vi "TCP Multiple Connections - Server.vi"() -> ()   [LabVIEW 2011]
doc: "This is the TCP server VI that supports multiple connections from client VIs."
panel:
  in  "Stop":bool
  out "Current Data":dbl
  out "# of Connections":i32
  # "Overview: Demonstrates the use of the TCP functions to initialize a TCP server that can send data to multiple client VIs.\nInstructions:\n1. Run the VI.\n2. Open TCP Multiple Connections - Client 1.vi and follow the instructions on its front panel.\n3. Open TCP Multiple Connections - Client 2.vi and follow the instructions on its front panel.\n4. Click Stop to stop the VI."
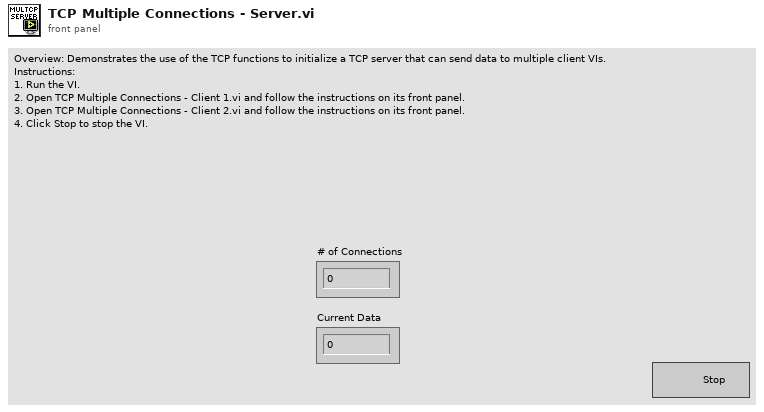
[diagram p1: front panel]
types:
  T1 = cluster{"Clients":refnum<k5>[], "Listener":refnum<k5>}
  T2 = enum16{"Initialize", "Status Check", "Send Data", "Stop"}
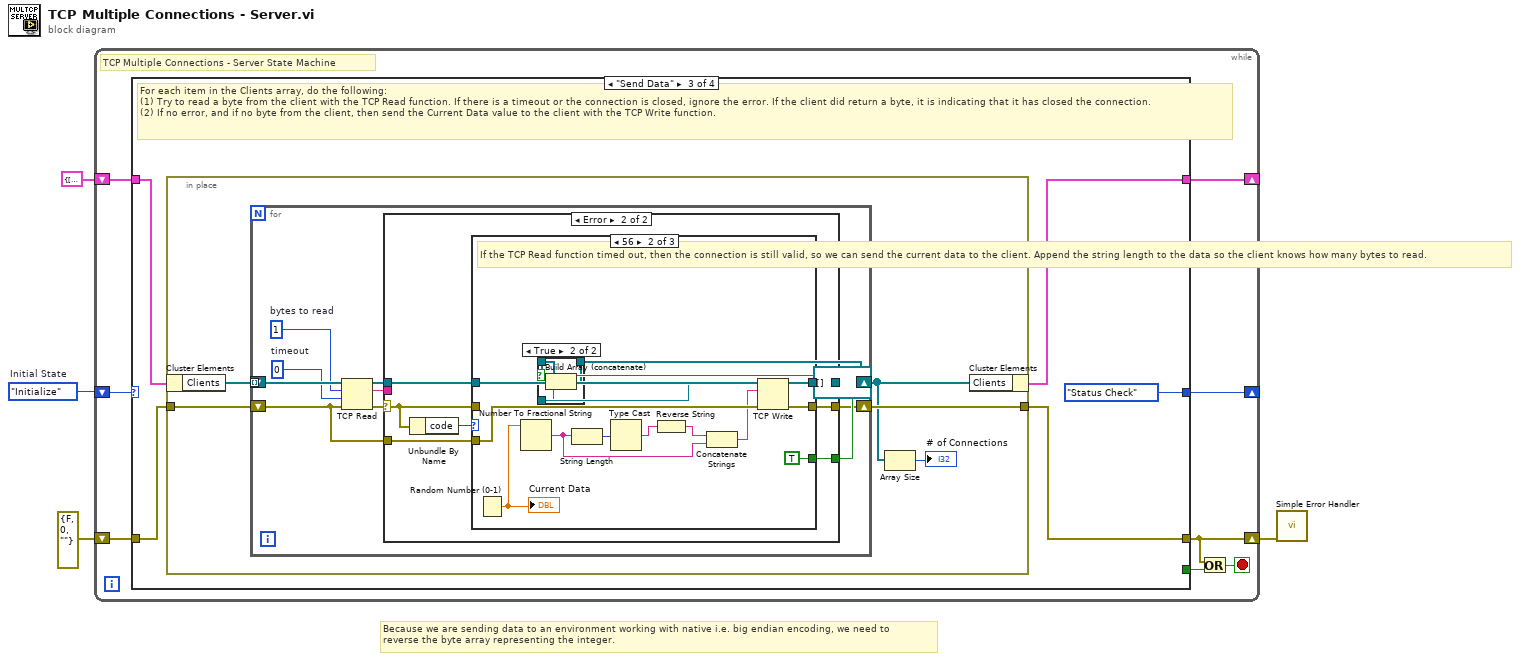
[diagram p0: block diagram]
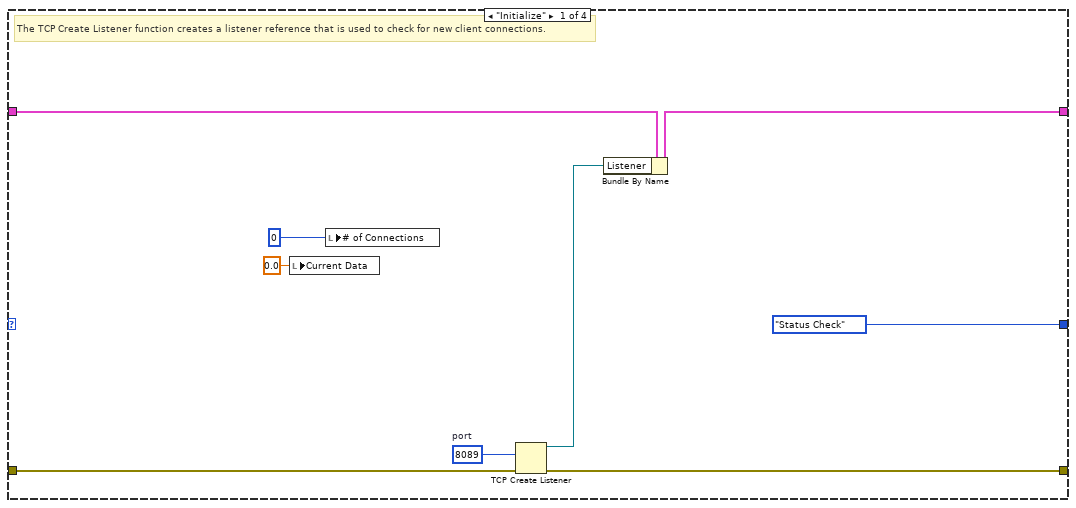
[diagram p2: hidden frame]
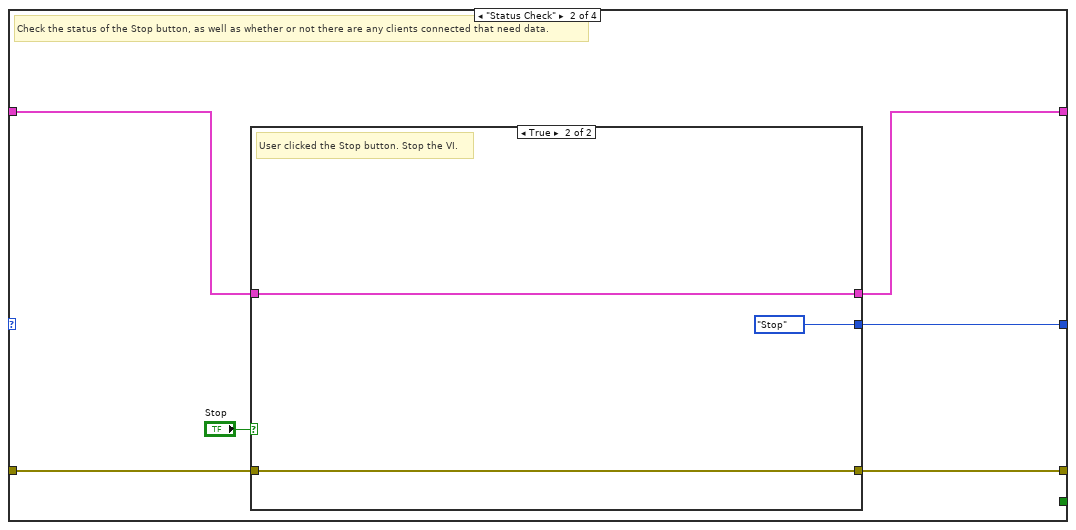
[diagram p3: hidden frame]
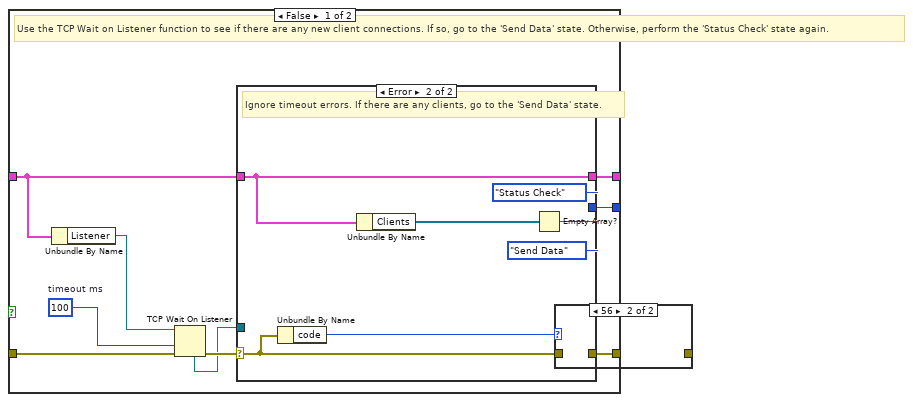
[diagram p4: hidden frame]
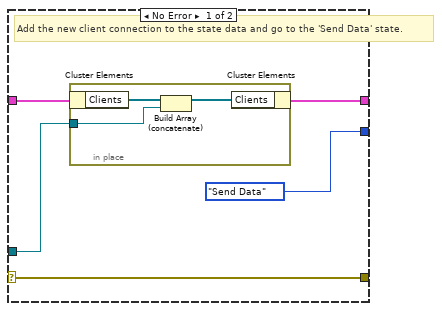
[diagram p5: hidden frame]
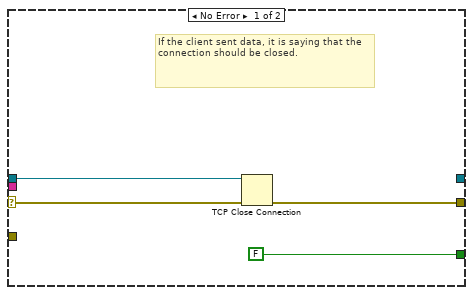
[diagram p8: hidden frame]
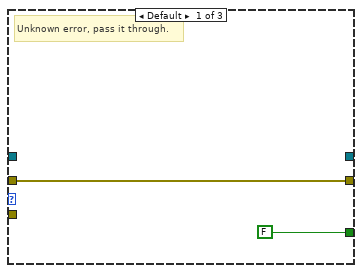
[diagram p9: hidden frame]
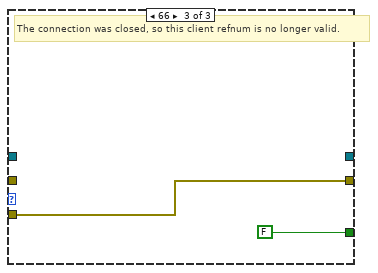
[diagram p10: hidden frame]
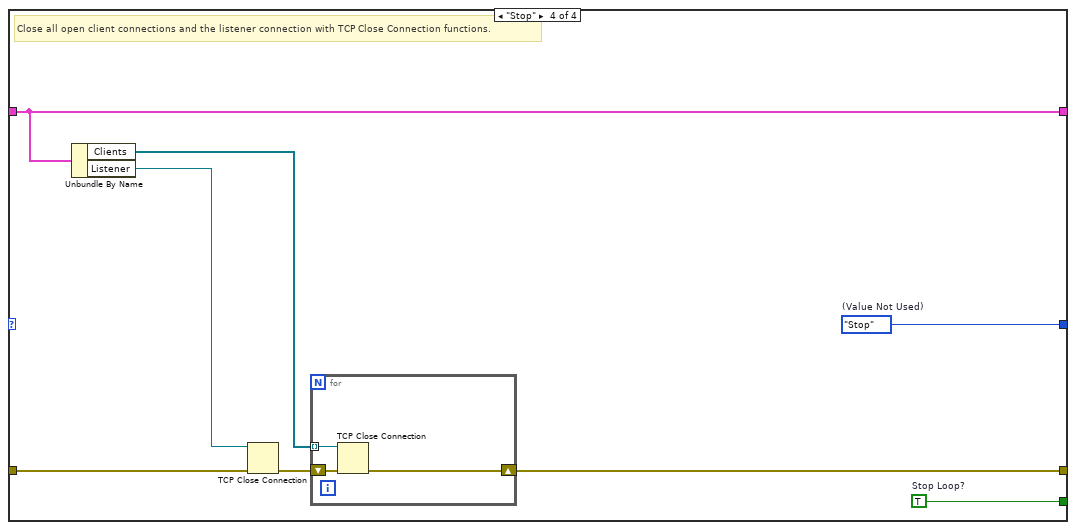
[diagram p11: hidden frame]
diagram:
  w4 = T2."Initialize"  # Initial State
  # "Because we are sending data to an environment working with native i.e. big endian encoding, we need to\nreverse the byte array representing the integer."
  n1 = while {
    shift-right: [w11] -> _
    shift-left: w4 -> [w12]
    shift-right: [w9] -> _
    shift-left: T1 {"Clients"=[], "Listener"=refnum} ("Data") -> [w10]
    shift-right: [w5] -> w1
    shift-left: errorcluster {"status"=FALSE, "code"=0, "source"=""} ("error constant") -> [w8]
    stop <- w6 stop-if-true
    # "TCP Multiple Connections - Server State Machine"
    n2 = case shown="\"Send Data\"" w12 {
      tunnel: [T2."Status Check" ("States") w27 T2."Status Check" ("States") w112] -> w11
      tunnel: [_ _ _ w119] -> w7
      tunnel: w10 -> [w19 w23 w61 w118]
      tunnel: [w18 w22 w60 w118] -> w9
      tunnel: w8 -> [w21 w26 w63 w117]
      tunnel: [w20 w25 w62 w115] -> w5
      frame "Initialize" {
        w16 = u16 8089  # port
        # "The TCP Create Listener function creates a listener reference that is used to check for new client connections."
        n3 = local write "Current Data"(0.0 ("Current Data")) -> ()
        n4 = local write "# of Connections"(0 ("Number of Client Connections")) -> ()
        n5 = TCP Create Listener(8:w21, 10:w16) -> (0:w20:errorcluster, 3:w17:refnum<k5>)  [unwired: 4 out]
        n6 = Bundle By Name(cluster=w19, "Listener"=w17) -> (w18:T1)
      }
      frame "Status Check" {
        # "Check the status of the Stop button, as well as whether or not there are any clients connected that need data."
        n7 = case shown="True" "Stop" {
          tunnel: [w36 T2."Stop" ("States")] -> w27
          tunnel: w26 -> [w35 w58]
          tunnel: [w28 w58] -> w25
          tunnel: w23 -> [w31 w57]
          tunnel: [w30 w57] -> w22
          frame False {
            w34 = 100  # timeout ms
            # "Use the TCP Wait on Listener function to see if there are any new client connections. If so, go to the 'Send Data' state. Otherwise, perform the 'Status Check' state again."
            n8 = Unbundle By Name(w31) -> ("Listener"=w29:refnum<k5>)
            n9 = TCP Wait On Listener(8:w35, 9:w34, 11:w29) -> (0:w33:errorcluster, 4:w32:refnum<k5>)  [unwired: 4 out]
            n10 = case shown="Error" w33 {
              selector: w33 -> [w39 w53]
              tunnel: [T2."Send Data" ("States") w47] -> w36
              tunnel: w32 -> [w40 _]
              tunnel: w31 -> [w41 w50]
              tunnel: [w38 w50] -> w30
              tunnel: [w39 w51] -> w28
              frame No Error {
                # "Add the new client connection to the state data and go to the 'Send Data' state."
                n11 = in-place {
                  in-place-border: w40 -> [w42]
                  n12 = in-place-cluster #1(w41) -> ("Clients"=w44:refnum<k5>[])
                  n13 = Build Array (concatenate)(w44, w42) -> (w43:refnum<k5>[])
                  n14 = in-place-cluster #1("Clients"=w43) -> (w38:T1)
                }
              }
              frame Error {
                # "Ignore timeout errors. If there are any clients, go to the 'Send Data' state."
                n15 = Unbundle By Name(w53) -> ("code"=w52:i32)
                n16 = Unbundle By Name(w50) -> ("Clients"=w49:refnum<k5>[])
                n17 = Empty Array?(array=w49) -> (empty?=w48:bool)
                n18 = case shown="56" w52 {
                  tunnel: w53 -> [w54 _]
                  tunnel: [w54 w55] -> w51
                  frame Default {
                  }
                  frame 56 {
                    w55 = errorcluster {"status"=FALSE, "code"=0, "source"=""}  # no error
                  }
                }
                n19 = Select(t=T2."Status Check" ("States"), s=w48, f=T2."Send Data" ("States")) -> (s? t:f=w47:T2)
              }
            }
          }
          frame True {
            # "User clicked the Stop button. Stop the VI."
          }
        }
      }
      frame "Send Data" {
        # "For each item in the Clients array, do the following:\n(1) Try to read a byte from the client with the TCP Read function. If there is a timeout or the connection is closed, ignore the error. If the client did return a byte, it is indicating that it has closed the connection.\n(2) If no error, and if no byte from the client, then send the Current Data value to the client with the TCP Write function."
        n20 = in-place {
          in-place-border: w63 -> [w69]
          in-place-border: [w68] -> w62
          n21 = in-place-cluster #2(w61) -> ("Clients"=w66:refnum<k5>[])
          n22 = for {
            tunnel: w66 -> [w81] mode=indexing
            shift-right: [w73] -> w68
            shift-left: w69 -> [w72]
            shift-right: [w70] -> w65
            shift-left: refnum<k5>[] [] ("Array") -> [w71]
            w78 = 0  # timeout
            w79 = 1  # bytes to read
            n23 = TCP Read(connection ID=w81, bytes to read=w79, error in (no error)=w72, 9:w78) -> (connection ID out=w80:refnum<k5>, data out=w76:string, error out=w77:errorcluster)  [unwired: 1 out]
            n24 = case shown="Error" w77 {
              selector: w77 -> [w88 w95]
              tunnel: w80 -> [w89 w92]
              tunnel: w76 -> [_ _]
              tunnel: [_ w90] -> w75
              tunnel: [FALSE w91] -> w74
              tunnel: [w86 w94] -> w73
              tunnel: w72 -> [_ w93]
              frame No Error {
                # "If the client sent data, it is saying that the connection should be closed."
                # "If the client sent data, it is saying that the connection should be closed."
                n25 = TCP Close Connection(connection ID=w89, error in (no error)=w88) -> (error out=w86:errorcluster)  [unwired: 2 out]
              }
              frame Error {
                # "Ignore connection closed and timeout errors"
                n26 = Unbundle By Name(w95) -> ("code"=w96:i32)
                n27 = case shown="56" w96 {
                  tunnel: w95 -> [w98 _ _]
                  tunnel: [w98 w109 w111] -> w94
                  tunnel: w93 -> [_ w105 w111]
                  tunnel: w92 -> [_ w108 _]
                  tunnel: [FALSE TRUE FALSE] -> w91
                  tunnel: [_ w107 _] -> w90
                  frame Default {
                    # "Unknown error, pass it through."
                  }
                  frame 56 {
                    # "If the TCP Read function timed out, then the connection is still valid, so we can send the current data to the client. Append the string length to the data so the client knows how many bytes to read."
                    n28 = Random Number (0-1)() -> (number: 0 to 1=w104:dbl)
                    "Current Data" <- w104
                    n29 = Number To Fractional String(number=w104) -> (F-format string=w99:string)  [unwired: 3 in]
                    n30 = String Length(string=w99) -> (length=w103:i32)
                    n31 = Type Cast(x=w103) -> (*(type *) &x=w101:string)  [unwired: 1 in]
                    n32 = Reverse String(1:w101) -> (0:w100:string)
                    n33 = Concatenate Strings(w100, w99) -> (w102:string)
                    n34 = TCP Write(connection ID=w108, data in=w102, error in (no error)=w105) -> (connection ID out=w107:refnum<k5>, error out=w109:errorcluster)  [unwired: 2 out]
                  }
                  frame 66 {
                    # "The connection was closed, so this client refnum is no longer valid."
                  }
                }
              }
            }
            n35 = case shown="True" w74 {
              tunnel: w71 -> [w82 w84]
              tunnel: w75 -> [_ w83]
              tunnel: [w82 w85] -> w70
              frame False {
              }
              frame True {
                n36 = Build Array (concatenate)(w84, w83) -> (w85:refnum<k5>[])
              }
            }
          }
          n37 = Array Size(array=w65) -> (size(s)=→"# of Connections":i32)
          n38 = in-place-cluster #2("Clients"=w65) -> (w60:T1)
        }
      }
      frame "Stop" {
        w112 = T2."Stop"  # (Value Not Used)
        w119 = TRUE  # Stop Loop?
        # "Close all open client connections and the listener connection with TCP Close Connection functions."
        n39 = Unbundle By Name(w118) -> ("Clients"=w116:refnum<k5>[], "Listener"=w113:refnum<k5>)
        n40 = TCP Close Connection(connection ID=w113, error in (no error)=w117) -> (error out=w114:errorcluster)  [unwired: 1 in, 1 out]
        n41 = for {
          shift-right: [w121] -> w115
          shift-left: w114 -> [w122]
          tunnel: w116 -> [w120] mode=indexing
          n42 = TCP Close Connection(connection ID=w120, error in (no error)=w122) -> (error out=w121:errorcluster)  [unwired: 1 in, 1 out]
        }
      }
    }
    n43 = Or(x=w5, y=w7) -> (x .or. y?=w6:bool)
  }
  n44 = call <vilib>:"Simple Error Handler.vi"("error in (no error)"=w1) -> ()  [unwired: 4 in, 5 out]
